vi "Dashboard Main.vi"() -> ()   [LabVIEW 2014]
uses:
  <vilib>/event_ctls.llb/eventvkey.ctl
  <vilib>/Utility/config.llb/NI_LVConfig.lvlib
  <vilib>/Utility/config.llb/Write Key (I32).vi
  <vilib>/Rock Robotics/WPI/Dashboard/WPI_DashboardLogging Global.vi
  <vilib>/Utility/config.llb/Write Key (String).vi
  <vilib>/Rock Robotics/Network Tables/SD Read Number.vi
  <vilib>/Rock Robotics/Network Tables/SD Write Numeric Array.vi
panel:
  in  "TCP":refnum<k5>
  in  "Rec Mode":enum32{"Stop", "Record", "Playback"}(radio)
  in  "Vision":u16(ring) items=["Camera Off", "USB Camera SW", "USB Camera HW", "IP Camera"]
  out "Camera IP":string
  out "Image Message":string="Timeout in Camera Communications"
  in  "Dashboard Tab":T1(tab)
  out "Battery Meter":dbl(slide) scale=0.0..14.0 scale format="%#_2e"
  in  "Camera Settings":T2={"Frame Rate"=30, "Compression"=30, "Size"=1} {"Frame Rate" scale=1.0..30.0; "Size" items=["640x480", "320x240", "160x120"]}
  out "MotorChart R":cluster{"Numeric":dbl, "Numeric":dbl}(graph)
  out "MotorChart L":T3(graph)
  out "JS1 Z":dbl(slide) scale=-1.0..1.0 scale format="%#_2e"
  out "JS1 Graph":cluster{"X":dbl, "Y":dbl}[](graph)
  out "JS1 Buttons":T4
  out "JS2 Z":dbl(slide) scale=-1.0..1.0 scale format="%#_2e"
  out "JS2 Graph":cluster{"X":dbl, "Y":dbl}[](graph)
  out "JS2 Buttons":T4
  out "Mode":T5(ring)=enum."Auto Disabled"
  in  "DB Camera Config":bool
  out "fps":dbl format="%#.1g"
  out "Mbps":dbl format="%#.1g"
  out "Mbps 2":bool
  out "Robot Position":cluster{"Y":dbl[], "Y":dbl[]}[](graph)
  out "Gyro":dbl(knob) scale=0.0..360.0
  out "Distance from Object":dbl(knob) scale=0.1..100.0
  out "Arm":dbl(slide) max=6.0 scale=0.0..6.0 scale format="%.6g"
  out "Totes":u8(slide) scale=0.0..6.0
  in  "DB/String 9":string
  in  "DB/String 8":string
  in  "DB/String 7":string
  in  "DB/String 6":string
  in  "DB/String 5":string
  in  "DB/String 4":string
  in  "DB/String 3":string
  in  "DB/String 2":string
  in  "DB/String 1":string
  in  "DB/String 0":string
  in  "DB/Slider 0":dbl(slide) scale=0.0..5.0
  in  "DB/Slider 1":dbl(slide) scale=0.0..5.0
  in  "DB/Slider 2":dbl(slide) scale=0.0..5.0
  in  "DB/Slider 3":dbl(slide) scale=0.0..5.0
  out "DB/LED 3":bool
  out "DB/LED 2":bool
  out "DB/LED 1":bool
  out "DB/LED 0":bool
  in  "DB/Button 3":bool
  in  "DB/Button 2":bool
  in  "DB/Button 1":bool
  in  "DB/Button 0":bool caption="New Name"
  in  "Preset Auton Routine":T6(ring)
  in  "Action":T7(ring)
  out "X/Y/a Output":dbl[][](array[numeric]) caption="X pos     Y pos    Angle    Action"
  in  "If an object is detected...":T8(ring)
  in  "Input":dbl[](array[numeric])
  in  "Index No.":u8
  in  "Add Keyframe":bool
  in  "Remove Keyframe":bool
  in  "Load Preset":bool
  in  "Test Slider":dbl(slide) scale=0.0..100.0 scale format="%#_3g"
  in  "On/Off":bool caption="Solenoid"
  in  "Test Name":u16(ring) items=["Select the test to run...", "Example Test", "-------------------------------", "List of tests is built in robot code.", "Replace with your own automated tests."]
  in  "Test Tree":string(tree)
  in  "Motor":cluster{"Value":dbl, "Enable":bool} {"Value" scale=-1.0..1.0 scale format="%#_3g"}
  out "Progress":T9 {"Test Progress" scale=0.0..100.0}
  in  "Rev/Fwd":cluster{"Forward":bool, "Reverse":bool}
  in  "Test Ring":u16(ring) items=["Monochrome", "Color"]
  in  "Listbox":i32(listbox)
  out "Tree":string(tree)
  out "Camera Image":T10(plugin-control)
  out "Boolean":bool
  # "Left"
  # "Right"
  # "Batt"
  # "312"
  # "NOTE: Set Angle to -1 if you don't\nwant to reposition after movement.\nAngle relative to starting angle\n(unless gryo is present)"
  # "0"
  # "324"
  # "Values measured in inches"
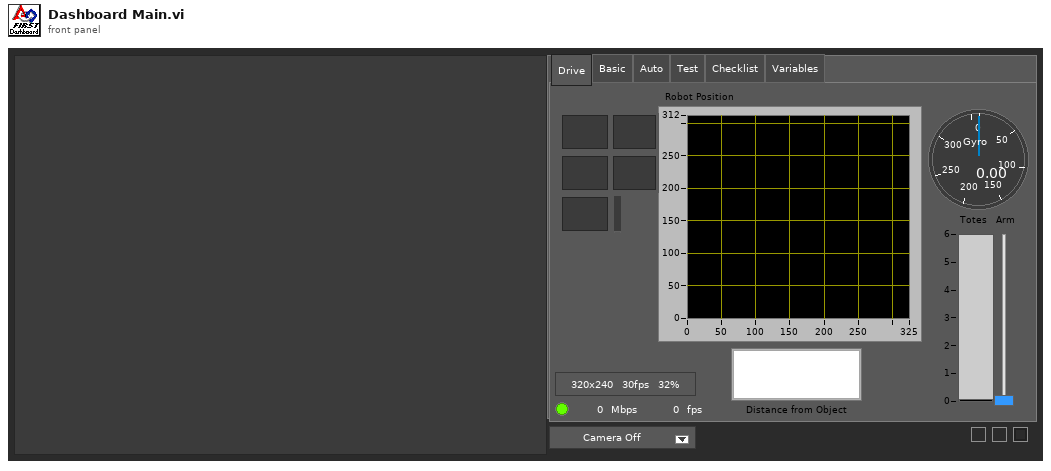
[diagram p1: front panel]
types:
  T1 = enum32{"Drive", "Basic", "Auto", "Test", "Checklist", "Variables"}
  T2 = cluster{"Frame Rate":i32, "Compression":i32, "Size":u16}
  T3 = cluster{"Numeric":dbl, "Numeric":dbl, "Battery V":dbl}
  T4 = cluster{bool, bool, bool, bool, bool, bool, bool, bool, bool, bool, bool, bool}
  T5 = enum8{"Tele-Op Disabled", "Tele-Op Enabled", "Auto Disabled", "Auto Enabled", "Test Disabled", "Test Enabled", "Disconnected", "No Code", "E-Stop"}
  T6 = enum8{"Score 3 Totes", "Move 1 Tote", "Score 3 Containers", "Move 1 Container", "Move 1 Tote & Container", "Get Center Step Containers", "Get Left Step Container", "Get Right Step Containter", "Custom..."}
  T7 = enum16{"Do Nothing", "Get Tote ", "Get Tote w/ Arms", "Get Container w/ Arms", "Stack Tote", "Place Object on Ground", "Eject Tote"}
  T8 = enum8{"Pick up (tote)", "Pick up (container)", "Avoid", "Wait until clear"}
  T9 = cluster{"Test Progress":u8, "Test Progress Text":string}
  T10 = typedef "IMAQ Image.ctl" = refnum<image>
  T11 = enum32{"Drive", "Basic", "Custom", "Test", "Checklist", "Variables"}
  T12 = typedef "Image Type" = u32
  T13 = cluster{"Camera Image":refnum<vi>, "Dashboard Tab":refnum<vi>, "Boolean":refnum<vi>, "Vision":refnum<vi>, "Rec Mode":refnum<vi>, "Test Slider":refnum<vi>, "On/Off ":refnum<vi>, "Test Ring":refnum<vi>, "Rev/Fwd":refnum<vi>, "Test Name":refnum<vi>, "Motor":refnum<vi>, "Progress":refnum<vi>, "CheckList":refnum<vi>, "Tree":refnum<vi>, "Test Tree":refnum<vi>}
  T14 = cluster{"Error Strings":string, "Disable Counts":cluster{u16, u16}, "Rail Faults":cluster{u16, u16, u16}, "Robot IP":string, "DB Mode":u8, "Event Info":cluster{"Name":string, "Type":u8, "Number":u16, "Replay":u8}, "Camera Addr":string}
  T15 = cluster{"Storage":cluster{"Disk Free":u64, "RAM Block":u32, "RAM free":u32}, "CPU Utilization":cluster{"CPU % ISR":sgl, "CPU % Time Crit":sgl, "CPU % Timed Str":sgl, "CPU % High":sgl, "CPU % Above":sgl, "CPU % Normal":sgl, "CPU % Low":sgl}, "CAN":cluster{"% Bus Utilization":sgl, "Bus Off Cnt":u32, "TX_FIFO Full Cnt":u32, "Receive Error Cnt":u8, "Transmit Error Cnt":u8}, "HID":cluster{"HID Outputs":u32, "Rumble Low":u16, "Rumble High":u16}[]}
  T16 = cluster{"Status bits":cluster{"Test Mode":bool, "Autonomous":bool, "Enabled":bool, "Code Start":bool, "Brownout":bool, "Reserved 2":bool, "Reserved 3":bool, "E-Stop":bool}, "Code Trace":cluster{"Disabled":bool, "TeleOp":bool, "Auto":bool, "Test":bool}, "Controller Type":enum16{"unknown", "cRIO", "roboRio"}, "Code?":enum16{"unknown", "noCode", "code"}, "Battery V":dbl}
  T17 = cluster{"Control Bits":cluster{"TestMode":bool, "Autonomous":bool, "Enabled":bool, "FMS Present":bool, bool, bool, bool, "E-Stop":bool}, "Team Station ":u8, "Countdown":sgl, "Joystick Values":cluster{"Axes":dbl[], "Buttons":bool[], "POVs":i16[]}[]}
  T18 = cluster{"Axes":dbl[], "Buttons":bool[], "POVs":i16[]}[]
  T19 = cluster{"[0]":i16, "[1]":i16, "[2]":i16, "[3]":i16, "[4]":i16, "[5]":i16, "[6]":i16, "[7]":i16, "[8]":i16}
  T20 = cluster{"Axes":dbl[], "Buttons":bool[], "POVs":i16[]}
  T21 = cluster{"Buttons[0]":bool, "Buttons[1]":bool, "Buttons[2]":bool, "Buttons[3]":bool, "Buttons[4]":bool, "Buttons[5]":bool, "Buttons[6]":bool, "Buttons[7]":bool, "Buttons[8]":bool, "Buttons[9]":bool, "Buttons[10]":bool, "Buttons[11]":bool}
  T22 = typedef "NI_LVConfig.lvlib/Config Data RefNum.ctl" = refnum<k1>
  T23 = cluster{"Operation":enum16{"Update", "Clear"}, "Color Box":u32}[]
  T24 = typedef "eventvkey.ctl" = enum16{"ASCII", "Enter", "Return", "Shift", "Ctrl", "Alt", "Cmd", "Opt", "Caps", "NumLock", "Clear", "Break", "Up", "Down", "Left", "Right", "Insert", "Delete", "Home", "End", "PageUp", "PageDown", "Escape", "Help", "Pause", "ScrollLock", "F1", "F2", "F3", "F4", "F5", "F6", "F7", "F8", "F9", "F10", "F11", "F12", "F13", "F14", "F15", "F16", "F17", "F18", "F19", "F20", "F21", "F22", "F23", "F24", "Play", "VolumeUp", "VolumeDown", "Mute", "Two Byte Char"}
  T25 = cluster{"Image Size":bool, "Image Type":bool, "Pixel Value":bool, "ROI Information":bool, "Zoom Factor":bool}
  T26 = enum8{"Enabled", "Disabled", "Disabled and Grayed Out"}
  T27 = cluster{"Operation":enum16{"Update", "Clear"}, "Color Box":u32}
  T28 = cluster{"Add Keyframe":bool, "Remove Keyframe":bool, "Load Preset":bool}
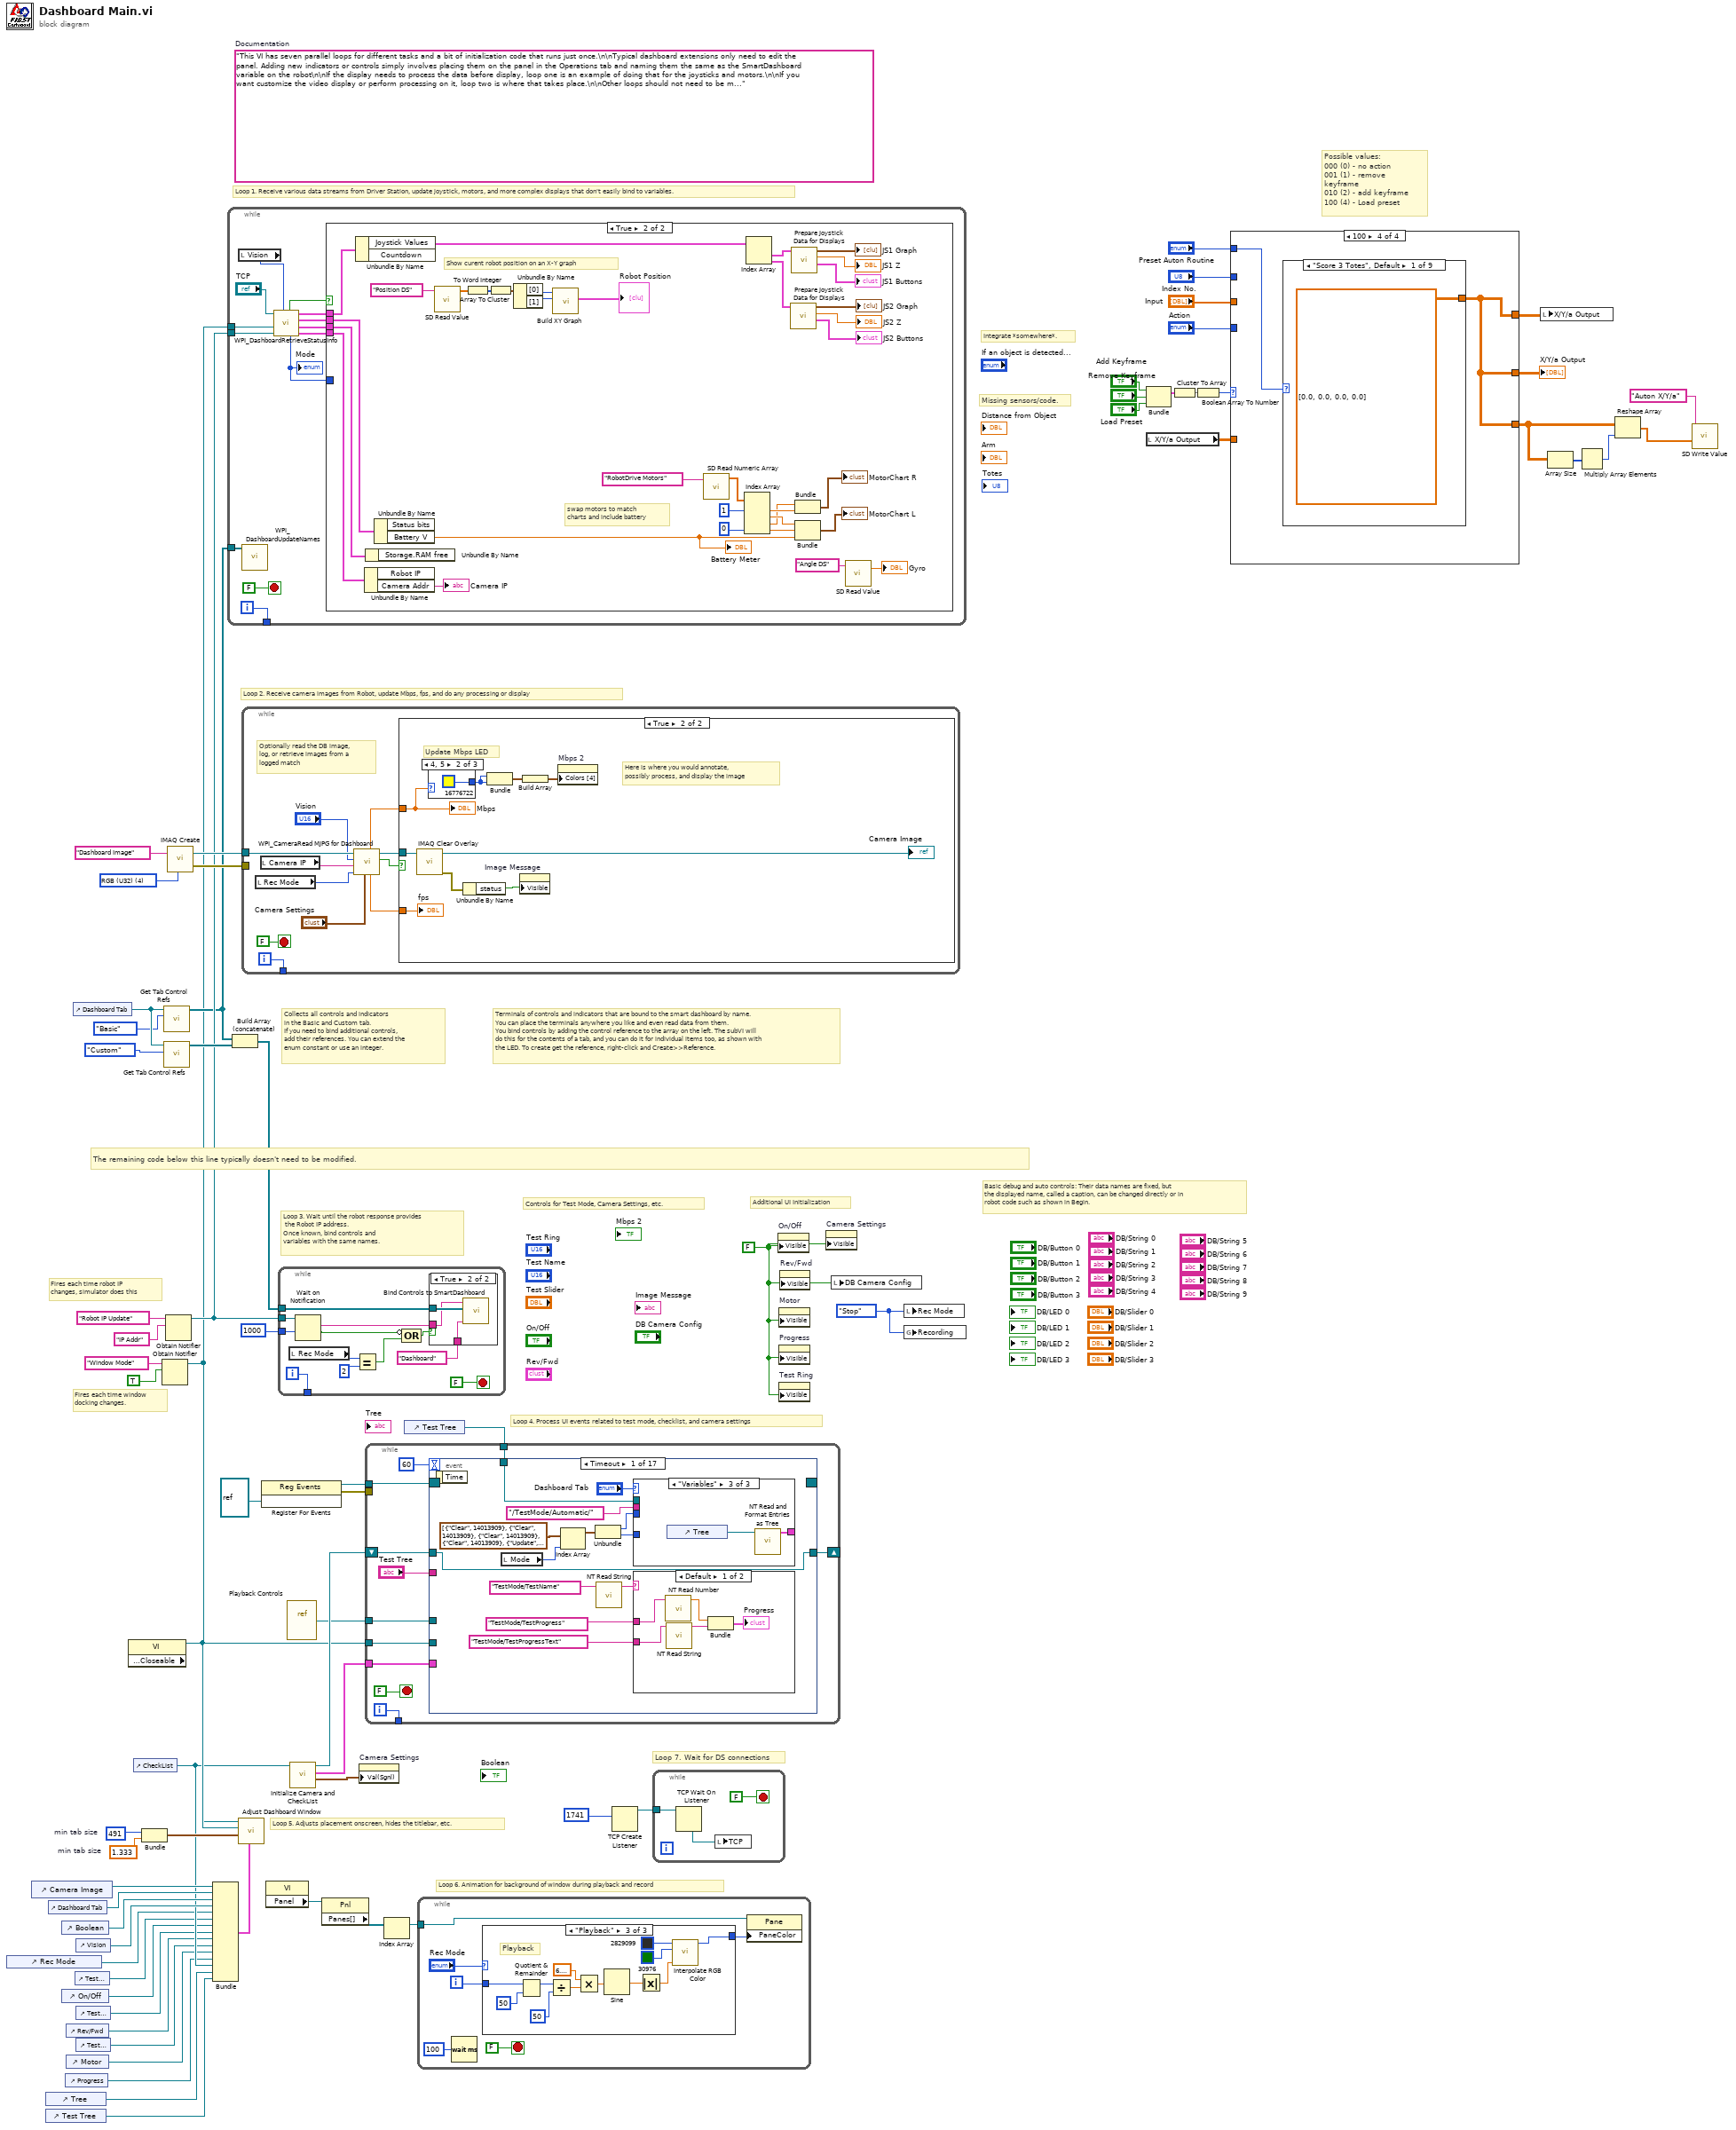
[diagram p0: block diagram]
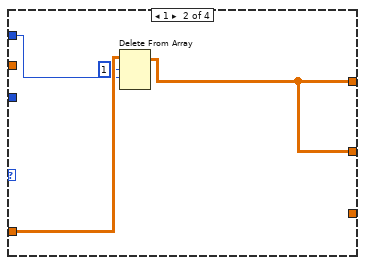
[diagram p3: hidden frame]
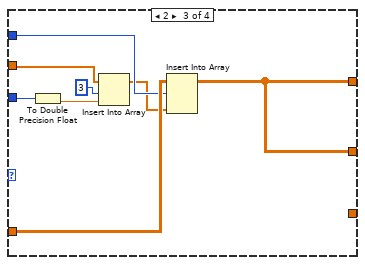
[diagram p4: hidden frame]
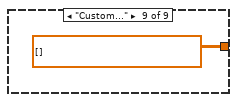
[diagram p12: hidden frame]
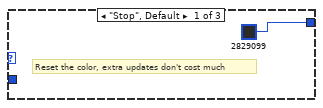
[diagram p14: hidden frame]
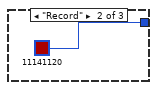
[diagram p15: hidden frame]
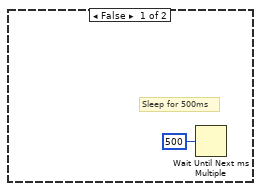
[diagram p17: hidden frame]
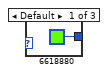
[diagram p18: hidden frame]
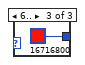
[diagram p19: hidden frame]
diagram:
  w42 = 491  # min tab size
  w41 = 1.333  # min tab size
  w50 = enum32{"Stop", "Record", "Playback"}."Stop" ("Rec Mode")
  w24 = FALSE ("Visible")
  (unwired) "This VI has seven parallel loops for different tasks and a bit of initialization code that runs just once.\n\nTypical dashboard extensions only need to edit the panel. Adding new indicators or controls simply involves placing them on the panel in the Operations tab and naming them the same as the SmartDashboard variable on the robot\n\nIf the display needs to process the data before display, loop one is an example of doing that for the joysticks and motors.\n\nIf you want customize the video display or perform processing on it, loop two is where that takes place.\n\nOther loops should not need to be modified. They are pretty standard, and document the task they perform."  # Documentation
  w70 = T12 4 items=["Grayscale (U8)", "Grayscale (I16)", "Grayscale (SGL)", "Complex (CSG)", "RGB (U32)", "HSL (U32)", "RGB (U64)"] ("Image Type")
  # "Possible values:\n000 (0) - no action\n001 (1) - remove keyframe\n010 (2) - add keyframe\n100 (4) - Load preset"
  # "Integrate *somewhere*."
  # "Missing sensors/code."
  # "Loop 7. Wait for DS connections"
  # "Basic debug and auto controls: Their data names are fixed, but\nthe displayed name, called a caption, can be changed directly or in\nrobot code such as shown in Begin."
  # "Controls for Test Mode, Camera Settings, etc."
  # "Additional UI Initialization"
  # "Loop 6. Animation for background of window during playback and record"
  # "Fires each time robot IP\nchanges, simulator does this"
  # "Fires each time window\ndocking changes."
  # "Collects all controls and indicators\nin the Basic and Custom tab.\nIf you need to bind additional controls,\nadd their references. You can extend the\nenum constant or use an integer."
  # "The remaining code below this line typically doesn't need to be modified."
  # "Loop 4. Process UI events related to test mode, checklist, and camera settings"
  # "Terminals of controls and indicators that are bound to the smart dashboard by name.\nYou can place the terminals anywhere you like and even read data from them.\nYou bind controls by adding the control reference to the array on the left. The subVI will\ndo this for the contents of a tab, and you can do it for individual items too, as shown with\nthe LED. To create get the reference, right-click and Create>>Reference."
  # "Loop 3. Wait until the robot response provides\n the Robot IP address.\nOnce known, bind controls and\nvariables with the same names."
  # "Loop 5. Adjusts placement onscreen, hides the titlebar, etc."
  # "Loop 1. Receive various data streams from Driver Station, update joystick, motors, and more complex displays that don't easily bind to variables."
  # "Loop 2. Receive camera images from Robot, update Mbps, fps, and do any processing or display"
  n1 = control-ref of="Rec Mode"() -> (w30:refnum<vi>)
  n2 = control-ref of="Camera Image"() -> (w45:refnum<vi>)
  n3 = control-ref of="Tree"() -> (w34:refnum<vi>)
  n4 = control-ref of="Test Tree"() -> (w33:refnum<vi>)
  n5 = control-ref of="Dashboard Tab"() -> (w44:refnum<vi>)
  n6 = control-ref of="Boolean"() -> (w39:refnum<vi>)
  n7 = control-ref of="On/Off"() -> (w28:refnum<vi>)
  n8 = control-ref of="Progress"() -> (w25:refnum<vi>)
  n9 = control-ref of="Rev/Fwd"() -> (w26:refnum<vi>)
  n10 = control-ref of="Motor"() -> (w31:refnum<vi>)
  n11 = control-ref of="Dashboard Tab"() -> (w48:refnum<vi>)
  n12 = control-ref of="Test Slider"() -> (w29:refnum<vi>)
  n13 = control-ref of="Vision"() -> (w43:refnum<vi>)
  n14 = control-ref of="Test Ring"() -> (w27:refnum<vi>)
  n15 = control-ref of="Test Name"() -> (w32:refnum<vi>)
  n16 = property class="VI" props=["Front Panel.Closeable"]() -> (reference out=w49:refnum<vi>)  [unwired: 2 in, 2 out]
  n17 = control-ref of="CheckList"() -> (w35:refnum<vi>)
  n18 = Bundle("min tab size"=w42, "min tab size"=w41) -> (w40:cluster{"min tab size":i32, "min tab size":dbl})  [unwired: 1 in]
  n19 = Obtain Notifier(name (unnamed)="Window Mode", notification data type=TRUE) -> (notifier out=w21:refnum<notifier>)  [unwired: 2 in, 2 out]
  n20 = call <vilib>:"Get Tab Control Refs.vi"("Page Index"=T11."Basic" ("Dashboard Tab"), "TabControl in"=w48) -> ("ControlsOnPage"=w22:refnum<vi>[])  [unwired: 9 in]
  n21 = call <vilib>:"Get Tab Control Refs.vi"("Page Index"=T11."Custom" ("Dashboard Tab"), "TabControl in"=w48) -> ("ControlsOnPage"=w47:refnum<vi>[])  [unwired: 9 in]
  n22 = Obtain Notifier(name (unnamed)="Robot IP Update", notification data type="IP Addr" ("name (unnamed)")) -> (notifier out=w23:refnum<notifier>)  [unwired: 2 in, 2 out]
  n23 = call "IMAQ Create"("Image Name"="Dashboard Image", "Image Type"=w70) -> ("New Image"=w68:T10, "error out"=w67:errorcluster)  [unwired: 2 in, 1 out]
  n24 = Bundle("Camera Image"=w45, "Dashboard Tab"=w44, "Boolean"=w39, "Vision"=w43, "Rec Mode"=w30, "Test Slider"=w29, "On/Off"=w28, "Test Ring"=w27, "Rev/Fwd"=w26, "Test Name"=w32, "Motor"=w31, "Progress"=w25, "CheckList"=w35, "Tree"=w34, "Test Tree"=w33) -> (w36:T13)  [unwired: 1 in]
  n25 = while {
    tunnel: [w82] -> _
    tunnel: w23 -> [w76]
    tunnel: w22 -> [w75]
    tunnel: w21 -> [w71]
    i -> [w82]
    stop <- FALSE stop-if-true
    n26 = local read "Vision"() -> (w73:u16)
    n27 = call <vilib>:"WPI_DashboardUpdateNames.vi"("Controls on Tab"=w75) -> ()  [unwired: 11 in]
    n28 = call <vilib>:"WPI_DashboardRetrieveStatusInfo.vi"("Vision"=w73, "Binding Refnum"=w76, "Window Mode Notifier"=w71, "TCP Cnx"="TCP") -> ("Power and Errors"=w77:T14, "Robot Metrics"=w80:T15, "Status Info"=w81:T16, "Control Info"=w78:T17, "Robot Mode"=w74:T5, "Process?"=w79:bool)  [unwired: 2 in]
    "Mode" <- w74
    n29 = case shown="True" w79 {
      tunnel: w81 -> [_ w117]
      tunnel: w80 -> [_ w116]
      tunnel: w78 -> [_ w115]
      tunnel: w77 -> [_ w114]
      tunnel: w74 -> [_ _]
      frame False {
      }
      frame True {
        # "Show curent robot position on an X-Y graph"
        # "swap motors to match\ncharts and include battery"
        n30 = Unbundle By Name(w115) -> ("Joystick Values"=w103:T18)  [unwired: 1 out]
        n31 = Unbundle By Name(w114) -> ("Camera Addr"=→"Camera IP":string)  [unwired: 1 out]
        n32 = Unbundle By Name(w116) -> ()  [unwired: 1 out]
        n33 = Unbundle By Name(w117) -> ("Battery V"=w84:dbl)  [unwired: 1 out]
        "Battery Meter" <- w84
        n34 = call-poly <vilib>:"SD Read Value.vi"("Name"="Position DS") -> ("Numeric Array"=w89:dbl[])  [unwired: 8 in, 2 out]
        n35 = To Word Integer(number=w89) -> (16bit integer=w88:i16[])
        n36 = Array To Cluster(array=w88) -> (cluster=w87:T19)
        n37 = Unbundle By Name(w87) -> ("[0]"=w86:i16, "[1]"=w85:i16)
        n38 = call "Build XY Graph"("Y Input"=w85, "X Input"=w86) -> ("XY Graph"=→"Robot Position":cluster{"X":dbl[], "Y":dbl[]}[])  [unwired: 8 in, 1 out]
        n39 = call <vilib>:"SD Read Numeric Array.vi"("Name"="RobotDrive Motors") -> ("Numeric Array"=w105:dbl[])  [unwired: 8 in, 2 out]
        n40 = Index Array(array=w105, index #1=1, index #4=0) -> (element #1=w109:dbl, element #2=w110:dbl, element #3=w108:dbl, element #4=w113:dbl)  [unwired: 2 in]
        n41 = Index Array(array=w103) -> (element #1=w102:T20, element #2=w97:T20)  [unwired: 2 in]
        n42 = call "Prepare Joystick Data for Displays.vi"("Joystick Values"=w97) -> ("Buttons"=→"JS2 Buttons":T21, "Z Axis"=→"JS2 Z":dbl, "Cartesian Data"=→"JS2 Graph":cluster{"X axis":dbl, "X axis":dbl}[])  [unwired: 8 in]
        n43 = call "Prepare Joystick Data for Displays.vi"("Joystick Values"=w102) -> ("Buttons"=→"JS1 Buttons":T21, "Z Axis"=→"JS1 Z":dbl, "Cartesian Data"=→"JS1 Graph":cluster{"X axis":dbl, "X axis":dbl}[])  [unwired: 8 in]
        n44 = Bundle("Numeric"=w108, "Numeric"=w109) -> (→"MotorChart R":cluster{"Numeric":dbl, "Numeric":dbl})  [unwired: 1 in]
        n45 = Bundle("Numeric"=w110, "Numeric"=w113, "Battery V"=w84) -> (→"MotorChart L":T3)  [unwired: 1 in]
        n46 = call-poly <vilib>:"SD Read Value.vi"("Name"="Angle DS") -> ("Numeric"=→"Gyro":dbl)  [unwired: 8 in, 2 out]
      }
    }
  }
  n47 = Build Array (concatenate)(w22, w47) -> (w46:refnum<vi>[])
  n48 = call "Adjust Dashboard Window.vi"("Sizing Refnums"=w36, "Size Constraints"=w40, "VI"=w49, "Notifier in"=w21) -> ()  [unwired: 8 in]
  n49 = while {
    tunnel: w68 -> [w126]
    tunnel: w67 -> [_]
    tunnel: [w127] -> _
    i -> [w127]
    stop <- FALSE stop-if-true
    # "Optionally read the DB image,\nlog, or retrieve images from a\nlogged match"
    n50 = local read "Rec Mode"() -> (w120:enum32{"Stop", "Record", "Playback"})
    n51 = local read "Camera IP"() -> (w118:string)
    n52 = call <vilib>:"WPI_CameraRead MJPG for Dashboard.vi"("Camera Settings"="Camera Settings", "Rec Mode"=w120, "Camera IP"=w118, "Camera Mode"="Vision", "Refnum in"=w126) -> ("Active"=w124:bool, "Refnum out"=w125:T10, "FPS"=w123:dbl, "Bandwidth (Mbps)"=w122:dbl)  [unwired: 3 in]
    n53 = case shown="True" w124 {
      tunnel: w125 -> [_ w133]
      tunnel: w122 -> [_ w132]
      tunnel: w123 -> [_ w130]
      frame False {
        # "Sleep for 500ms"
        n54 = Wait Until Next ms Multiple(millisecond multiple=u32 500) -> ()  [unwired: 1 out]
      }
      frame True {
        # "Here is where you would annotate,\npossibly process, and display the image"
        # "Update Mbps LED"
        n55 = call "IMAQ Clear Overlay"("Image"=w133) -> ("error out"=w137:errorcluster, "Image Out"=→"Camera Image":T10)  [unwired: 2 in, 7 out]
        n56 = case shown="4, 5" w132 {
          tunnel: [u32 6618880 ("Color Box") u32 16776722 ("Color Box") u32 16716800 ("Color Box")] -> w134
          frame Default {
          }
          frame 4, 5 {
          }
          frame 6.. {
          }
        }
        n57 = Unbundle By Name(w137) -> ("status"=w138:bool)
        n58 = Bundle("Color Box"=w134, "Color Box"=w134) -> (w136:cluster{"Color Box":u32, "Color Box":u32})  [unwired: 1 out]
        n59 = property on="Image Message" class="Str"("Visible"=w138) -> ()  [unwired: 2 in, 2 out]
        n60 = Build Array(w136) -> (w135:cluster{"Color Box":u32, "Color Box":u32}[])
        n61 = property on="Mbps 2" class="Bool (strict)"("Colors [4]"=w135) -> ()  [unwired: 2 in, 2 out]
        "Mbps" <- w132
        "fps" <- w130
      }
    }
  }
  n62 = register-events(refnum<vi> refnum) -> (reference out=w54:refnum<event-registration>, error out=w53:errorcluster)  [unwired: 2 in]
  n63 = property class="VI"() -> ("Panel"=w57:refnum<vi>)  [unwired: 2 in, 2 out]
  n64 = while {
    tunnel: w46 -> [w153]
    tunnel: w23 -> [w151]
    tunnel: [w149] -> _
    tunnel: u32 1000 ("milliseconds to wait") -> [w148]
    i -> [w149]
    stop <- FALSE stop-if-true
    n65 = local read "Rec Mode"() -> (w144:enum32{"Stop", "Record", "Playback"})
    n66 = Wait on Notification(notifier=w151, timeout in ms (-1)=w148) -> (notification=w150:string, timed out?=w146:bool)  [unwired: 2 in, 2 out]
    n67 = Equal?(x=w144, y=u16 2 ("Rec Mode")) -> (x = y?=w145:bool)
    n68 = Compound Arithmetic op=OR(invert w146, w145) -> (w147:bool)
    n69 = case shown="True" w147 {
      tunnel: w153 -> [_ w156]
      tunnel: w150 -> [_ w155]
      tunnel: "Dashboard" -> [_ w154]
      frame False {
      }
      frame True {
        n70 = call <vilib>:"Bind Controls to SmartDashboard.vi"("Client Name"=w154, "Bound Control Refs"=w156, "Server IP Address"=w155) -> ()  [unwired: 9 in]
      }
    }
  }
  n71 = vi-ref "Playback Controls.vi"() -> (w55:refnum<vi>)
  n72 = call "Initialize Camera and CheckList.vi"("ListBox in"=w35) -> ("Cluster"=w61:cluster{"value":i32, "value":i32, "index":i32}, "Array"=w62:cluster{string[]}[], "File Refnum"=w60:T22)  [unwired: 8 in]
  n73 = property class="Pnl"(reference=w57) -> ("Panes[]"=w58:refnum<vi>[])  [unwired: 1 in, 2 out]
  n74 = property on="Camera Settings" class="Clust (strict)"("Val(Sgnl)"=w61) -> ()  [unwired: 2 in, 2 out]
  n75 = Index Array(array=w58) -> (element=w56:refnum<vi>)  [unwired: 1 in]
  n76 = control-ref of="Test Tree"() -> (w59:refnum<vi>)
  n77 = while {
    tunnel: w62 -> [w164]
    shift-right: [w163] -> _
    shift-left: w60 -> [w162]
    tunnel: [w161] -> _
    tunnel: w59 -> [w160]
    tunnel: w55 -> [w159]
    tunnel: w54 -> [w158]
    tunnel: w53 -> [_]
    tunnel: w49 -> [w157]
    i -> [w161]
    stop <- FALSE stop-if-true
    n78 = event shown="[0] Timeout" {
      selector: w158 -> [_ _ _ _ _ _ _ _ _ _ _ _ _ _ _ _ _]
      dyn-events: [_ _ _ _ _ _ _ _ _ _ _ _ _ w402 _ _ _] -> _
      timeout: u32 60 ("milliseconds to wait") -> [_ _ _ _ _ _ _ _ _ _ _ _ _ _ _ _ _]
      tunnel: w160 -> [w176 _ _ _ _ _ _ _ _ _ _ _ _ _ _ _ _]
      tunnel: "Test Tree" -> [_ _ _ _ _ _ _ _ w371 w379 w381 w385 w393 _ _ _ _]
      tunnel: w164 -> [_ w198 _ _ _ _ w335 w365 _ _ _ _ _ _ _ _ _]
      tunnel: [w172 w197 w296 w301 w309 w321 w334 w358 w370 w377 w380 w384 w392 w404 w418 w419 w429] -> w163
      tunnel: w162 -> [w172 w197 w296 w301 w309 w321 w333 w358 w370 w377 w380 w384 w392 w404 w418 w419 w429]
      tunnel: w159 -> [_ _ _ _ _ _ _ _ _ _ _ _ _ w405 _ w422 _]
      tunnel: w157 -> [_ _ _ _ _ _ _ _ _ _ _ _ _ w400 _ _ _]
      event Timeout {
        n79 = event-data() -> ()  [unwired: 1 in, 1 out]
        n80 = local read "Mode"() -> (w175:T5)
        n81 = Index Array(array=T23 [{"Operation"=enum."Clear", "Color Box"=14013909}, {"Operation"=enum."Clear", "Color Box"=14013909}, {"Operation"=enum."Clear", "Color Box"=14013909}, {"Operation"=enum."Clear", "Color Box"=14013909}, {"Operation"=enum."Update", "Color Box"=14013909}, {"Operation"=enum."Update", "Color Box"=16777215}, {"Operation"=enum."Clear", "Color Box"=14013909}, {"Operation"=enum."Clear", "Color Box"=14013909}, {"Operation"=enum."Clear", "Color Box"=14013909}], index=w175) -> (element=w170:T27)
        n82 = Unbundle(w170) -> ("Operation"=w169:enum16{"Update", "Clear"}, "Color Box"=w168:u32)
        n83 = call <vilib>:"NT Read String.vi"("Name"="TestMode/TestName") -> ("String"=w179:string)  [unwired: 9 in, 1 out]
        n84 = case shown="\"Variables\"" "Dashboard Tab" {
          tunnel: w176 -> [_ w187 _]
          tunnel: "/TestMode/Automatic/" ("Name Pattern") -> [_ w186 _]
          tunnel: w169 -> [_ w185 _]
          tunnel: [_ _ w189] -> _
          tunnel: w168 -> [_ w181 _]
          frame "Auto", Default {
          }
          frame "Test" {
            w184 = -2 ("Active Item:Row Number")
            n85 = call <vilib>:"NT Read and Format Entries as Tree.vi"("Operation"=w185, "Name Pattern"=w186, "Tree Refnum"=w187) -> ()  [unwired: 7 in, 2 out]
            n86 = property on="Test Tree" class="Tree (strict)"("Active Item Row Number"=w184, "ActiveColNum"=w184, "CellBG"=w181, "Active Item Row Number"=-1 ("Active Item:Row Number"), "CellBG"=u32 5789784 ("Color Box")) -> ()  [unwired: 2 in, 2 out]
          }
          frame "Variables" {
            n87 = control-ref of="Tree"() -> (w188:refnum<vi>)
            n88 = call <vilib>:"NT Read and Format Entries as Tree.vi"("Tree Refnum"=w188) -> ("Formatted Strings"=w189:cluster{"Name":string, "Value":string}[])  [unwired: 9 in, 1 out]
          }
        }
        n89 = case shown="Default" w179 {
          tunnel: "TestMode/TestProgress" ("Name") -> [w191 _]
          tunnel: "TestMode/TestProgressText" ("Name") -> [w190 _]
          frame Default {
            n90 = call <vilib>:"NT Read Number.vi"("Name"=w191) -> ("Numeric"=w192:dbl)  [unwired: 9 in, 1 out]
            n91 = call <vilib>:"NT Read String.vi"("Name"=w190) -> ("String"=w193:string)  [unwired: 9 in, 1 out]
            n92 = Bundle("Numeric"=w192, "String"=w193) -> (→"Progress":cluster{"Numeric":dbl, "String":string})  [unwired: 1 in]
          }
          frame "" {
            n93 = property on="Progress" class="Clust (strict)"("Visible"=FALSE) -> ()  [unwired: 2 in, 2 out]
            n94 = local write "Test Name"(u16 0) -> ()
          }
        }
      }
      event "Test Tree": Value Change {
        # "Show appropriate\ncontrols"
        n95 = event-data() -> ("CtlRef"=w201:refnum<vi>, "NewVal"=w199:string)  [unwired: 1 in]
        n96 = call <vilib>:"WPI_UtilitiesGetTreeIOName.vi"("NewVal"=w199, "TreeControl in"=w201) -> ("I/O Name"=w202:string)  [unwired: 9 in]
        n97 = case shown="\"Camera\"" w202 {
          selector: w202 -> [_ w209 _ w227 w236 _]
          tunnel: w199 -> [_ _ w224 w226 _ w243]
          tunnel: w198 -> [_ _ _ _ _ w242]
          frame Default {
            w204 = FALSE ("Visible")
            w203 = FALSE ("Visible")
            n98 = property on="Motor" class="Clust (strict)"("Visible"=w203) -> ()  [unwired: 2 in, 2 out]
            n99 = property on="Test Ring" class="Ring (strict)"("Visible"=w203) -> ()  [unwired: 2 in, 2 out]
            n100 = property on="Rev/Fwd" class="Clust (strict)"("Visible"=w204) -> ()  [unwired: 2 in, 2 out]
            n101 = property on="On/Off" class="Bool (strict)"("Visible"=w204) -> ()  [unwired: 2 in, 2 out]
            n102 = property on="Test Slider" class="Slide (strict)"("Visible"=w204) -> ()  [unwired: 2 in, 2 out]
          }
          frame "Motor", "PWM" {
            w210 = FALSE ("Visible")
            n103 = case shown="\"Motor\", Default" w209 {
              tunnel: [1.0 ("Value") -1.0 ("Value")] -> w208
              tunnel: [255.0 ("Value") 1.0 ("Value")] -> w207
              tunnel: [128.0 ("Value") 0.0 ("Value")] -> w206
              tunnel: [64.0 ("Value") 0.5 ("Value")] -> w205
              frame "PWM" {
              }
              frame "Motor", Default {
              }
            }
            n104 = property on="Motor" class="Clust (strict)"("Visible"=TRUE) -> ()  [unwired: 2 in, 2 out]
            n105 = property on="Value" class="Slide (strict)"("Value"=w206, "Scale.Minimum"=w208, "Scale.Maximum"=w207, "Scale.Increment"=w205) -> ()  [unwired: 2 in, 2 out]
            n106 = property on="On/Off" class="Bool (strict)"("Visible"=w210) -> ()  [unwired: 2 in, 2 out]
            n107 = property on="Test Slider" class="Slide (strict)"("Visible"=w210) -> ()  [unwired: 2 in, 2 out]
            n108 = property on="Test Ring" class="Ring (strict)"("Visible"=w210) -> ()  [unwired: 2 in, 2 out]
            n109 = property on="Rev/Fwd" class="Clust (strict)"("Visible"=w210) -> ()  [unwired: 2 in, 2 out]
          }
          frame "Servo" {
            w222 = FALSE ("Visible")
            n110 = call <vilib>:"NT Read Number.vi"("Name"=w224) -> ("Numeric"=w223:dbl)  [unwired: 9 in, 1 out]
            n111 = property on="Test Slider" class="Slide (strict)"("Visible"=TRUE, "Scale.Maximum"=170.0 ("Scale.Range:Maximum")) -> ()  [unwired: 2 in, 2 out]
            n112 = local write "Test Slider"(w223) -> ()
            n113 = property on="Motor" class="Clust (strict)"("Visible"=w222) -> ()  [unwired: 2 in, 2 out]
            n114 = property on="Rev/Fwd" class="Clust (strict)"("Visible"=w222) -> ()  [unwired: 2 in, 2 out]
            n115 = property on="On/Off" class="Bool (strict)"("Visible"=w222) -> ()  [unwired: 2 in, 2 out]
            n116 = property on="Test Ring" class="Ring (strict)"("Visible"=w222) -> ()  [unwired: 2 in, 2 out]
          }
          frame "Relay", "Solenoid" {
            w225 = FALSE ("Visible")
            n117 = property on="Motor" class="Clust (strict)"("Visible"=w225) -> ()  [unwired: 2 in, 2 out]
            n118 = property on="Test Slider" class="Slide (strict)"("Visible"=w225) -> ()  [unwired: 2 in, 2 out]
            n119 = Search and Replace String(input string=w226, search string="/Value  **", replace string="/Direction") -> (result string=w232:string)  [unwired: 5 in, 3 out]
            n120 = property on="Test Ring" class="Ring (strict)"("Visible"=w225) -> ()  [unwired: 2 in, 2 out]
            n121 = call <vilib>:"NT Read String.vi"("Name"=w232) -> ("String"=w230:string)  [unwired: 9 in, 1 out]
            n122 = Equal?(x="Both directions", y=w230) -> (x = y?=w228:bool)
            n123 = Not(x=w228) -> (.not. x?=w229:bool)
            n124 = property on="Rev/Fwd" class="Clust (strict)"("Visible"=w228) -> ()  [unwired: 2 in, 2 out]
            n125 = property on="On/Off" class="Bool (strict)"("Visible"=w229, "Caption.Text"=w227) -> ()  [unwired: 2 in, 2 out]
          }
          frame "Compressor", "Digital Out" {
            w235 = FALSE ("Visible")
            # "Get direction and finish"
            n126 = property on="Motor" class="Clust (strict)"("Visible"=w235) -> ()  [unwired: 2 in, 2 out]
            n127 = property on="Test Slider" class="Slide (strict)"("Visible"=w235) -> ()  [unwired: 2 in, 2 out]
            n128 = property on="Test Ring" class="Ring (strict)"("Visible"=w235) -> ()  [unwired: 2 in, 2 out]
            n129 = property on="On/Off" class="Bool (strict)"("Visible"=TRUE, "Caption.Text"=w236) -> ()  [unwired: 2 in, 2 out]
            n130 = property on="Rev/Fwd" class="Clust (strict)"("Visible"=FALSE) -> ()  [unwired: 2 in, 2 out]
          }
          frame "Camera" {
            n131 = call <vilib>:"Get Last Path Segment.vi"("String in"=w243) -> ("String out"=w244:string)  [unwired: 10 in]
            n132 = property on="On/Off" class="Bool (strict)"("Visible"=FALSE) -> ()  [unwired: 2 in, 2 out]
            n133 = property on="Motor" class="Clust (strict)"("Visible"=FALSE) -> ()  [unwired: 2 in, 2 out]
            n134 = property on="Rev/Fwd" class="Clust (strict)"("Visible"=FALSE) -> ()  [unwired: 2 in, 2 out]
            n135 = case shown="\"White Balance  **\"" w244 {
              tunnel: w243 -> [w250 w259 w268 w277 w286 _ w292]
              tunnel: w242 -> [w248 w256 w265 w274 w283 _ _]
              frame "Size  **" {
                n136 = Index Array(array=w248) -> (element=w247:cluster{string[]})  [unwired: 1 in]
                n137 = call <vilib>:"NT Read String.vi"("Name"=w250) -> ("String"=w249:string)  [unwired: 9 in, 1 out]
                n138 = Unbundle(w247) -> (w245:string[])
                n139 = Match First String(2:w245, 3:w249) -> (0:w246:i32)  [unwired: 1 out]
                n140 = property on="Test Ring" class="Ring (strict)"("Value"=w246, "Strings []"=w245) -> ()  [unwired: 2 in, 2 out]
                n141 = property on="Test Ring" class="Ring (strict)"("Visible"=TRUE) -> ()  [unwired: 2 in, 2 out]
                n142 = property on="Test Slider" class="Slide (strict)"("Visible"=FALSE) -> ()  [unwired: 2 in, 2 out]
              }
              frame "White Balance  **" {
                n143 = Index Array(array=w256, index=1) -> (element=w257:cluster{string[]})
                n144 = call <vilib>:"NT Read String.vi"("Name"=w259) -> ("String"=w258:string)  [unwired: 9 in, 1 out]
                n145 = Unbundle(w257) -> (w254:string[])
                n146 = Match First String(2:w254, 3:w258) -> (0:w253:i32)  [unwired: 1 out]
                n147 = property on="Test Ring" class="Ring (strict)"("Value"=w253, "Strings []"=w254) -> ()  [unwired: 2 in, 2 out]
                n148 = property on="Test Ring" class="Ring (strict)"("Visible"=TRUE) -> ()  [unwired: 2 in, 2 out]
                n149 = property on="Test Slider" class="Slide (strict)"("Visible"=FALSE) -> ()  [unwired: 2 in, 2 out]
              }
              frame "Exposure  **" {
                n150 = Index Array(array=w265, index=2) -> (element=w266:cluster{string[]})
                n151 = call <vilib>:"NT Read String.vi"("Name"=w268) -> ("String"=w267:string)  [unwired: 9 in, 1 out]
                n152 = Unbundle(w266) -> (w262:string[])
                n153 = Match First String(2:w262, 3:w267) -> (0:w263:i32)  [unwired: 1 out]
                n154 = property on="Test Ring" class="Ring (strict)"("Value"=w263, "Strings []"=w262) -> ()  [unwired: 2 in, 2 out]
                n155 = property on="Test Ring" class="Ring (strict)"("Visible"=TRUE) -> ()  [unwired: 2 in, 2 out]
                n156 = property on="Test Slider" class="Slide (strict)"("Visible"=FALSE) -> ()  [unwired: 2 in, 2 out]
              }
              frame "Exposure Priority  **" {
                n157 = Index Array(array=w274, index=3) -> (element=w275:cluster{string[]})
                n158 = call <vilib>:"NT Read String.vi"("Name"=w277) -> ("String"=w276:string)  [unwired: 9 in, 1 out]
                n159 = Unbundle(w275) -> (w271:string[])
                n160 = Match First String(2:w271, 3:w276) -> (0:w272:i32)  [unwired: 1 out]
                n161 = property on="Test Ring" class="Ring (strict)"("Value"=w272, "Strings []"=w271) -> ()  [unwired: 2 in, 2 out]
                n162 = property on="Test Ring" class="Ring (strict)"("Visible"=TRUE) -> ()  [unwired: 2 in, 2 out]
                n163 = property on="Test Slider" class="Slide (strict)"("Visible"=FALSE) -> ()  [unwired: 2 in, 2 out]
              }
              frame "Color Enable  **" {
                n164 = Index Array(array=w283, index=4) -> (element=w284:cluster{string[]})
                n165 = call <vilib>:"NT Read String.vi"("Name"=w286) -> ("String"=w285:string)  [unwired: 9 in, 1 out]
                n166 = Unbundle(w284) -> (w280:string[])
                n167 = Match First String(2:w280, 3:w285) -> (0:w281:i32)  [unwired: 1 out]
                n168 = property on="Test Ring" class="Ring (strict)"("Value"=w281, "Strings []"=w280) -> ()  [unwired: 2 in, 2 out]
                n169 = property on="Test Ring" class="Ring (strict)"("Visible"=TRUE) -> ()  [unwired: 2 in, 2 out]
                n170 = property on="Test Slider" class="Slide (strict)"("Visible"=FALSE) -> ()  [unwired: 2 in, 2 out]
              }
              frame Default {
                n171 = property on="Test Ring" class="Ring (strict)"("Visible"=FALSE) -> ()  [unwired: 2 in, 2 out]
                n172 = property on="Test Slider" class="Slide (strict)"("Visible"=FALSE) -> ()  [unwired: 2 in, 2 out]
              }
              frame "Brightness  **", "Color Level  **", "Compression  **", "FPS  **", "Sharpness  **" {
                n173 = call <vilib>:"NT Read Number.vi"("Name"=w292) -> ("Numeric"=w291:dbl)  [unwired: 9 in, 1 out]
                n174 = local write "Test Slider"(w291) -> ()
                n175 = property on="Test Ring" class="Ring (strict)"("Visible"=FALSE) -> ()  [unwired: 2 in, 2 out]
                n176 = property on="Test Slider" class="Slide (strict)"("Visible"=TRUE, "Scale.Maximum"=100.0 ("Scale.Range:Maximum")) -> ()  [unwired: 2 in, 2 out]
              }
            }
          }
        }
        n177 = property on="Progress" class="Clust (strict)"("Visible"=FALSE) -> ()  [unwired: 2 in, 2 out]
      }
      event "Test Name": Mouse Enter {
        # "Populate the ring with the list of tests"
        n178 = event-data() -> ()  [unwired: 1 in, 1 out]
        n179 = call <vilib>:"NT Read String Array.vi"("Name"="TestMode/TestList") -> ("String Array"=w300:string[])  [unwired: 9 in, 1 out]
        n180 = Build Array (concatenate)("Select the test to run...", w300) -> (w299:string[])
        n181 = property on="Test Name" class="Ring (strict)"("Strings []"=w299) -> ()  [unwired: 2 in, 2 out]
      }
      event "Test Name": Value Change {
        w302 = FALSE ("Visible")
        # "Tell the robot the test name to run"
        n182 = event-data() -> ("NewVal"=w306:u16)  [unwired: 1 in]
        n183 = property on="Test Name" class="Ring (strict)"() -> ("Strings []"=w307:string[])  [unwired: 2 in, 2 out]
        n184 = local write "Progress"(T9 {"Test Progress"=0, "Test Progress Text"=""} ("Progress")) -> ()
        n185 = Index Array(array=w307, index=w306) -> (element=w305:string)
        n186 = call <vilib>:"NT Write String.vi"("String"=w305, "Name"="TestMode/TestName") -> ()  [unwired: 9 in, 1 out]
        n187 = property on="Progress" class="Clust (strict)"("Visible"=TRUE) -> ()  [unwired: 2 in, 2 out]
        n188 = property on="Motor" class="Clust (strict)"("Visible"=w302) -> ()  [unwired: 2 in, 2 out]
        n189 = property on="Test Slider" class="Slide (strict)"("Visible"=w302) -> ()  [unwired: 2 in, 2 out]
        n190 = property on="On/Off" class="Bool (strict)"("Visible"=w302) -> ()  [unwired: 2 in, 2 out]
        n191 = property on="Rev/Fwd" class="Clust (strict)"("Visible"=w302) -> ()  [unwired: 2 in, 2 out]
        n192 = property on="Test Ring" class="Ring (strict)"("Visible"=w302) -> ()  [unwired: 2 in, 2 out]
      }
      event "Listbox": Double Click {
        # "Shift clears all"
        # "Update symbols on the listbox"
        n193 = event-data() -> ("PlatMods.Shift"=w310:bool, "Row"=w312:i32)  [unwired: 1 in]
        n194 = case shown="True" w310 {
          tunnel: w312 -> [w316 _]
          tunnel: 1 -> [w315 _]
          frame False {
            n195 = property on="Listbox" class="LstBox (strict)"() -> ("Item Symbols"=w314:i32[])  [unwired: 2 in, 2 out]
            n196 = Replace Array Subset(array=w314, new element=w315, index=w316) -> (w313:i32[])
            n197 = property on="Listbox" class="LstBox (strict)"("Item Symbols"=w313) -> ()  [unwired: 2 in, 2 out]
          }
          frame True {
            w317 = 0 ("Top Row")
            n198 = property on="Listbox" class="LstBox (strict)"() -> ("Number of Rows"=w319:u32)  [unwired: 2 in, 2 out]
            n199 = Initialize Array(0, w319) -> (w318:i32[])
            n200 = property on="Listbox" class="LstBox (strict)"("Top Row"=w317, "Value"=w317, "Item Symbols"=w318) -> ()  [unwired: 2 in, 2 out]
          }
        }
      }
      event "Listbox": Key Down {
        # "Update symbols on the listbox\nLeft and right keys check and uncheck"
        n201 = event-data() -> ("VKey"=w323:T24)  [unwired: 1 in]
        n202 = case shown="\"Left\", \"Right\"" w323 {
          selector: w323 -> [w328 _]
          tunnel: eventvkey."Left" ("VKey") -> [w326 _]
          frame "Left", "Right" {
            n203 = Equal?(x=w326, y=w328) -> (x = y?=w327:bool)
            n204 = Select(t=0, s=w327, f=1) -> (s? t:f=w329:i32)
            n205 = property on="Listbox" class="LstBox (strict)"() -> ("Item Symbols"=w332:i32[])  [unwired: 2 in, 2 out]
            n206 = Replace Array Subset(array=w332, new element=w329, index="Listbox") -> (w331:i32[])
            n207 = property on="Listbox" class="LstBox (strict)"("Item Symbols"=w331) -> ()  [unwired: 2 in, 2 out]
          }
          frame Default {
          }
        }
      }
      event "DB Camera Config": Value Change {
        # "Show or hide the cluster of controls, store in ini file"
        n208 = event-data() -> ("NewVal"=w336:bool)  [unwired: 1 in]
        n209 = case shown="False" w336 {
          tunnel: w335 -> [w345 _]
          tunnel: [w338 w356] -> w334
          tunnel: w333 -> [w337 w356]
          frame False {
            w352 = "Camera"
            w355 = FALSE ("Visible")
            n210 = local read "Camera Settings"() -> (w344:T2)
            n211 = Index Array(array=w345) -> (element=w348:cluster{string[]})  [unwired: 1 in]
            n212 = Unbundle(w344) -> ("Frame Rate"=w343:i32, "Compression"=w342:i32, "Size"=w346:u16)
            n213 = Unbundle(w348) -> (w347:string[])
            n214 = Index Array(array=w347, index=w346) -> (element=w341:string)
            n215 = call-poly <vilib>:"Write Key.vi"("section"=w352, "value"=w341, "key"="Size", "refnum"=w337) -> ("refnum out"=w354:T22)  [unwired: 2 in, 5 out]
            n216 = call-poly <vilib>:"Write Key.vi"("section"=w352, "value"=w343, "key"="FrameRate", "refnum"=w354) -> ("refnum out"=w353:T22)  [unwired: 1 in, 6 out]
            n217 = property on="Camera Settings" class="Clust (strict)"("Visible"=w355) -> ()  [unwired: 2 in, 2 out]
            n218 = local write "DB Camera Config"(w355) -> ()
            n219 = call-poly <vilib>:"Write Key.vi"("section"=w352, "value"=w342, "key"="Compression", "refnum"=w353) -> ("refnum out"=w339:T22)  [unwired: 1 in, 6 out]
            n220 = call <vilib>:"Close Config Data.vi"("refnum"=w339) -> ("file path"=w340:path)  [unwired: 2 in, 8 out]
            n221 = call <vilib>:"Open Config Data.vi"("configuration file path"=w340) -> ("refnum"=w338:T22)  [unwired: 8 in, 2 out]
          }
          frame True {
            n222 = property on="Camera Settings" class="Clust (strict)"("Visible"=TRUE) -> ()  [unwired: 2 in, 2 out]
          }
        }
      }
      event "Camera Settings": Value Change {
        # "Update summary string when any elements of DB camera change"
        n223 = event-data() -> ("NewVal"=w369:T2)  [unwired: 1 in]
        n224 = Index Array(array=w365) -> (element=w364:cluster{string[]})  [unwired: 1 in]
        n225 = Unbundle(w369) -> ("Frame Rate"=w360:i32, "Compression"=w359:i32, "Size"=w362:u16)
        n226 = Unbundle(w364) -> (w363:string[])
        n227 = Index Array(array=w363, index=w362) -> (element=w361:string)
        n228 = Format Into String(format string="%s   %dfps   %d%%", w361, w360, w359) -> (resulting string=w366:string)  [unwired: 2 in, 1 out]
        n229 = Build Array(w366) -> (w367:string[])
        n230 = property on="DB Camera Config" class="Bool (strict)"("Strings [4]"=w367) -> ()  [unwired: 2 in, 2 out]
      }
      event "Motor.Enable": Value Change {
        # "When the test mode otor enable helper is set, update that\ntree row item's value"
        n231 = event-data() -> ("NewVal"=w375:bool)  [unwired: 1 in]
        n232 = Unbundle("Motor") -> ("Value"=w374:dbl)  [unwired: 1 out]
        n233 = Select(t=w374, s=w375, f=0.0) -> (s? t:f=w372:dbl)
        n234 = call <vilib>:"NT Write Number.vi"("Numeric"=w372, "Name"=w371) -> ()  [unwired: 9 in, 1 out]
      }
      event "Test Slider": Value Change {
        # "When the test mode slider helper is set, update that\ntree row item's value"
        n235 = event-data() -> ("NewVal"=w378:dbl)  [unwired: 1 in]
        n236 = call <vilib>:"NT Write Number.vi"("Numeric"=w378, "Name"=w379) -> ()  [unwired: 9 in, 1 out]
      }
      event "On/Off": Value Change {
        # "When the test mode on/off helper value is set, update that\ntree row item's value"
        n237 = event-data() -> ("NewVal"=w383:bool)  [unwired: 1 in]
        n238 = Boolean To (0,1)(Boolean=w383) -> (0, 1=w382:i16)
        n239 = call <vilib>:"NT Write Number.vi"("Numeric"=w382, "Name"=w381) -> ()  [unwired: 9 in, 1 out]
      }
      event "Rev/Fwd": Value Change {
        # "When the test mode helper value for relays is set, update that\ntree row item's value"
        n240 = event-data() -> ("NewVal.Forward"=w391:bool, "NewVal.Reverse"=w390:bool)  [unwired: 1 in]
        n241 = Boolean To (0,1)(Boolean=w391) -> (0, 1=w387:i16)
        n242 = Boolean To (0,1)(Boolean=w390) -> (0, 1=w389:i16)
        n243 = Negate(x=w389) -> (-x=w388:i16)
        n244 = Add(x=w387, y=w388) -> (x+y=w386:i16)
        n245 = call <vilib>:"NT Write Number.vi"("Numeric"=w386, "Name"=w385) -> ()  [unwired: 9 in, 1 out]
      }
      event "Test Ring": Value Change {
        # "When a test mode helper value is selected from the ring,\nset the tree item's variable to the string value"
        n246 = event-data() -> ("NewVal"=w395:u16)  [unwired: 1 in]
        n247 = property on="Test Ring" class="Ring (strict)"() -> ("Strings []"=w396:string[])  [unwired: 2 in, 2 out]
        n248 = Index Array(array=w396, index=w395) -> (element=w394:string)
        n249 = call <vilib>:"NT Write String.vi"("String"=w394, "Name"=w393) -> ()  [unwired: 9 in, 1 out]
      }
      event "Rec Mode": Value Change {
        # "Update globals for recording mode and path to read log from.\nClear when logging and let NetworkTables set path for vision to\nuse."
        n250 = event-data() -> ("NewVal"=w406:enum32{"Stop", "Record", "Playback"})  [unwired: 1 in]
        n251 = case shown="\"Playback\"" w406 {
          tunnel: w405 -> [_ w408 w416]
          tunnel: [_ _ w415] -> w402
          tunnel: [_ _ w414] -> _
          tunnel: w400 -> [_ _ w412]
          tunnel: cluster{i32, i32} {-250, 170} -> [_ _ w411]
          tunnel: [_ _ T25 {"Image Size"=TRUE, "Image Type"=TRUE, "Pixel Value"=TRUE, "ROI Information"=TRUE, "Zoom Factor"=FALSE} ("Image Information Shown:All Elements")] -> w398
          tunnel: [_ _ TRUE ("Zoom Factor")] -> w397
          frame Default {
          }
          frame "Stop", "Record" {
            # "Place Window too"
            n252 = invoke class="VI" method="FP.Close"(reference=w408) -> (reference out=w407:refnum<vi>)  [unwired: 2 in, 2 out]
            n253 = invoke class="VI" method="Abort VI"(reference=w407) -> ()  [unwired: 2 in, 3 out]
          }
          frame "Playback" {
            n254 = call "Open Playback Panel.vi"("Offset"=w411, "DB VI Ref"=w412, "Playback in"=w416) -> ("Playback out"=w413:refnum<vi>)  [unwired: 8 in]
            n255 = register-events(w413) -> (reference out=w415:refnum<event-registration>, error out=w414:errorcluster)  [unwired: 2 in]
          }
        }
        n256 = global write "WPI_DashboardLogging Global.vi" "Recording"(w406) -> ()
        n257 = global write "WPI_DashboardLogging Global.vi" "Logging Filename"(path "") -> ()
        n258 = property on="Camera Image"("Image Information Shown"=w398, "Image Information Visible"=w397) -> ()  [unwired: 2 in, 2 out]
        n259 = call <vilib>:"WPI_DashboardNT Log FieldName Cache.vi"("Operation"=enum16{"Lookup/Add", "Index", "Clear"}."Clear") -> ()  [unwired: 8 in, 3 out]
      }
      event Panel Close {
        w417 = enum32{"Stop", "Record", "Playback"}."Stop" ("Rec Mode")
        # "Playback window has been closed, abort"
        n260 = event-data() -> ()  [unwired: 1 in, 4 out]
        n261 = local write "Rec Mode"(w417) -> ()
        n262 = global write "WPI_DashboardLogging Global.vi" "Recording"(w417) -> ()
      }
      event Panel Close {
        # "Abort playback window and ourself"
        n263 = event-data() -> ()  [unwired: 1 in, 4 out]
        n264 = invoke class="VI" method="FP.Close"(reference=w422) -> (reference out=w421:refnum<vi>)  [unwired: 2 in, 2 out]
        n265 = invoke class="VI" method="Abort VI"(reference=w421) -> (error out=w420:errorcluster)  [unwired: 2 in, 2 out]
        n266 = invoke class="VI" method="Abort VI"(error in=w420) -> ()  [unwired: 2 in, 3 out]
      }
      event "Vision": Value Change {
        # "Enable/Disable Compression slider.\nHW USB is hard-coded into the camera"
        n267 = event-data() -> ("NewVal"=w428:u16)  [unwired: 1 in]
        n268 = Equal?(x=w428, y=u32 2 ("milliseconds to wait")) -> (x = y?=w426:bool)
        n269 = Select(t=T26."Disabled and Grayed Out" ("Disabled"), s=w426, f=T26."Enabled" ("Disabled")) -> (s? t:f=w423:T26)
        n270 = property on="Compression" class="Slide (strict)"("DisabledEnum"=w423) -> ()  [unwired: 2 in, 2 out]
      }
    }
  }
  n271 = while {
    tunnel: w56 -> [w431]
    i -> [w434]
    stop <- FALSE stop-if-true
    n272 = Wait (ms)(milliseconds to wait=u32 100) -> ()  [unwired: 1 out]
    n273 = case shown="\"Playback\"" "Rec Mode" {
      tunnel: w434 -> [_ _ w449]
      tunnel: [u32 2829099 ("Base Color") u32 11141120 ("Target Color") w438] -> w430
      frame "Stop", Default {
        # "Reset the color, extra updates don't cost much"
      }
      frame "Record" {
      }
      frame "Playback" {
        # "Playback"
        n274 = Quotient & Remainder(x=w449, y=u32 50 ("milliseconds to wait")) -> (x-y*floor(x/y)=w445:u32)  [unwired: 1 out]
        n275 = Divide(x=w445, y=u32 50 ("milliseconds to wait")) -> (x/y=w442:dbl)
        n276 = Multiply(x=6.283185307179586, y=w442) -> (x*y=w447:dbl)
        n277 = Sine(x=w447) -> (sin(x)=w446:dbl)
        n278 = Absolute Value(x=w446) -> (abs(x)=w439:dbl)
        n279 = call "Interpolate RGB Color.vi"("Proportion"=w439, "Target Color"=u32 30976, "Base Color"=u32 2829099) -> ("Result Color"=w438:u32)  [unwired: 8 in]
      }
    }
    n280 = property class="Pane"(reference=w431, "PaneColor"=w430) -> ()  [unwired: 1 in, 2 out]
  }
  n281 = TCP Create Listener(10:u16 1741 ("timeout ms (25000)")) -> (3:w19:refnum<k5>)  [unwired: 4 in, 2 out]
  n282 = while {
    tunnel: w19 -> [w451]
    stop <- FALSE stop-if-true
    n283 = TCP Wait On Listener(11:w451) -> (4:w450:refnum<k5>)  [unwired: 3 in, 4 out]
    n284 = local write "TCP"(w450) -> ()
  }
  n285 = property on="On/Off" class="Bool (strict)"("Visible"=w24) -> ()  [unwired: 2 in, 2 out]
  n286 = property on="Motor" class="Clust (strict)"("Visible"=w24) -> ()  [unwired: 2 in, 2 out]
  n287 = property on="Progress" class="Clust (strict)"("Visible"=w24) -> ()  [unwired: 2 in, 2 out]
  n288 = property on="Test Ring" class="Ring (strict)"("Visible"=w24) -> ()  [unwired: 2 in, 2 out]
  n289 = property on="Rev/Fwd" class="Clust (strict)"("Visible"=w24) -> ()  [unwired: 2 in, 2 out]
  n290 = property on="Camera Settings" class="Clust (strict)"("Visible"=w24) -> ()  [unwired: 2 in, 2 out]
  n291 = local write "DB Camera Config"(w24) -> ()
  n292 = local write "Rec Mode"(w50) -> ()
  n293 = global write "WPI_DashboardLogging Global.vi" "Recording"(w50) -> ()
  n294 = Bundle("Add Keyframe"="Add Keyframe", "Remove Keyframe"="Remove Keyframe", "Load Preset"="Load Preset") -> (w16:T28)  [unwired: 1 in]
  n295 = local read "X/Y/a Output"() -> (w8:dbl[][])
  n296 = Cluster To Array(cluster=w16) -> (array=w15:bool[])
  n297 = Boolean Array To Number(Boolean array=w15) -> (number=w14:u32)
  n298 = case shown="100" w14 {
    tunnel: "Index No." -> [_ w455 w459 _]
    tunnel: "Input" -> [_ _ w464 _]
    tunnel: "Action" -> [_ _ w461 _]
    tunnel: [_ w453 w457 w465] -> w10
    tunnel: [_ w453 w457 w465] -> w9
    tunnel: w8 -> [_ w456 w460 _]
    tunnel: "Preset Auton Routine" -> [_ _ _ w466]
    tunnel: [_ _ _ w465] -> w5
    frame 0, Default {
      # "[do nothing]"
    }
    frame 1 {
      n299 = Delete From Array(array=w456, length=1, index (row)=w455) -> (array with subset deleted=w453:dbl[][])  [unwired: 1 in, 1 out]
    }
    frame 2 {
      n300 = To Double Precision Float(number=w461) -> (double precision float=w462:dbl)
      n301 = Insert Into Array(array=w464, index=3, new element=w462) -> (w458:dbl[])
      n302 = Insert Into Array(array=w460, index (row)=w459, new element=w458) -> (w457:dbl[][])  [unwired: 1 in]
    }
    frame 4 {
      n303 = case shown="\"Score 3 Totes\", Default" w466 {
        tunnel: [dbl[][] [[0.0, 0.0, 0.0, 0.0]] _ _ _ _ _ _ _ dbl[][] []] -> w465
        frame "Score 3 Totes", Default {
        }
        frame "Move 1 Tote" {
        }
        frame "Score 3 Containers" {
        }
        frame "Move 1 Container" {
        }
        frame "Move 1 Tote & Container" {
        }
        frame "Get Center Step Containers" {
        }
        frame "Get Left Step Container" {
        }
        frame "Get Right Step Containter" {
        }
        frame "Custom..." {
        }
      }
    }
  }
  "X/Y/a Output" <- w10
  n304 = local write "X/Y/a Output"(w9) -> ()
  n305 = Array Size(array=w5) -> (size(s)=w4:i32[])
  n306 = Multiply Array Elements(1:w4) -> (0:w3:i32)
  n307 = Reshape Array(w5, w3) -> (w2:dbl[])
  n308 = call-poly <vilib>:"SD Write Value.vi"("Numeric Array"=w2, "Name"="Auton X/Y/a") -> ()  [unwired: 8 in, 2 out]
